vi "Download_Folder_Prompt.vi"(10 "default name":string, 11 "DataCluster":T1) -> (2 "cancled?":bool, 3 "DataCluster out":T1)   [LabVIEW 2022 SP3]
uses:
  DataCluster.ctl
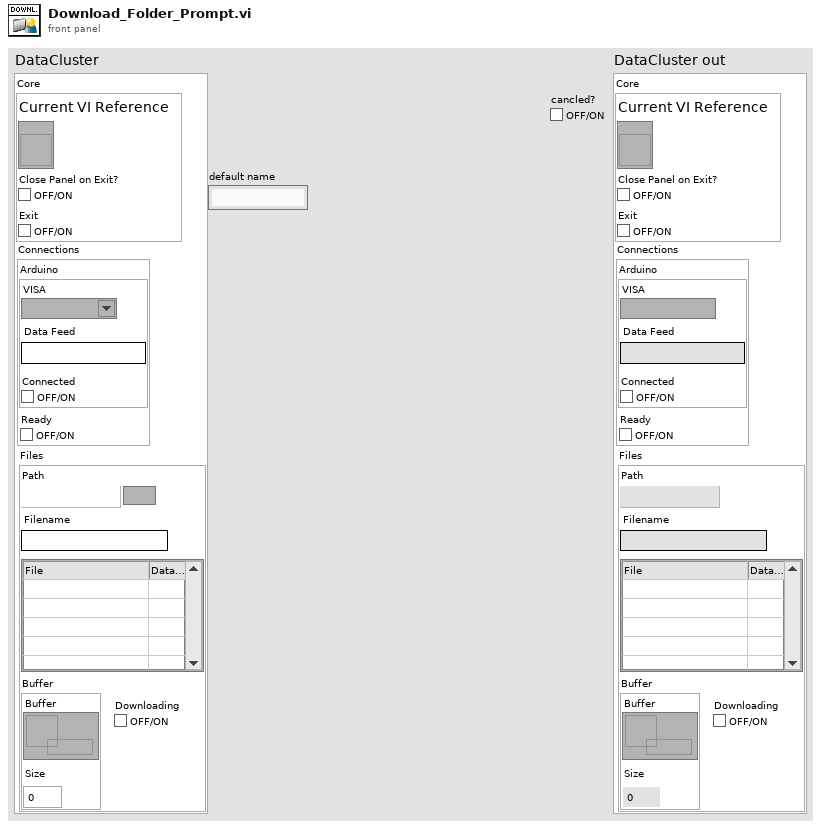
[diagram p1: front panel]
types:
  T1 = typedef "DataCluster.ctl" = cluster{"Core":cluster{"Current VI Reference":refnum<vi>, "Close Panel on Exit?":bool, "Exit":bool}, "Connections":cluster{"Arduino":cluster{"VISA":refnum<visa-resource-name>, "Data Feed":string, "Connected":bool}, "Ready":bool}, "Files":cluster{"Path":path, "Filename":string, "File List":i32, "Buffer":cluster{"Buffer":refnum<queue>, "Size":i32}, "Downloading":bool}}
  T2 = enum16{"open", "replace", "create", "open or create", "replace or create", "replace or create with confirmation"}
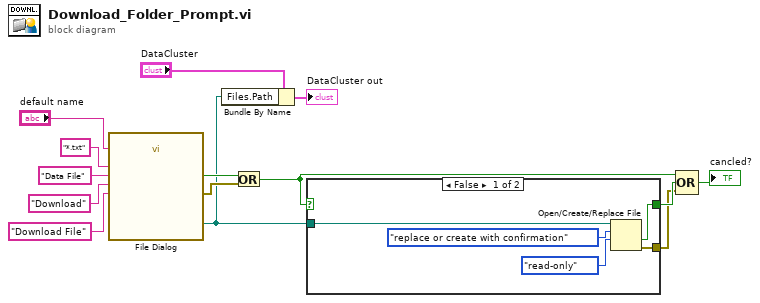
[diagram p0: block diagram]
diagram:
  n1 = call "File Dialog"("prompt"="Download File", "button label"="Download", "default name"="default name", "pattern (all files)"="*.txt", "pattern label"="Data File") -> ("selected path"=w4:path, "cancelled"=w13:bool, "error out"=w14:errorcluster)  [unwired: 7 in, 1 out]
  n2 = Bundle By Name(cluster="DataCluster", "Files.Path"=w4) -> (→"DataCluster out":T1)
  n3 = Or(x=w13, y=w14) -> (x .or. y?=w5:bool)
  n4 = case shown="False" w5 {
    selector: w5 -> [_ w20]
    tunnel: w4 -> [w19 _]
    tunnel: [w16 w20] -> w2
    tunnel: [w15 _] -> w1
    frame False {
      n5 = Open/Create/Replace File(file path (use dialog)=w19, operation (0:open)=T2."replace or create with confirmation", access (0:read/write)=enum16{"read/write", "read-only", "write-only"}."read-only") -> (cancelled=w16:bool, error out=w15:errorcluster)  [unwired: 3 in, 1 out]
    }
    frame True {
    }
  }
  n6 = Compound Arithmetic op=OR(w5, w2, w1) -> (→"cancled?":bool)
